vi "Draw_Grid_Over_Img.vi"(6 "[IN] Color":u32(colorbox)=16711680, 8 "error IN":errorcluster, 9 "[IN] Vertical step":i32=1 min=1 max=10000 step=1, 10 "[IN] Horiz step":i32=1 min=1 max=10000 step=1, 11 "[IN] Image":T1) -> (0 "error OUT":errorcluster, 3 "[OUT] Image":T1)   [LabVIEW 2020]
uses:
  <vilib>/vision/Image Controls.llb/IMAQ Image.ctl
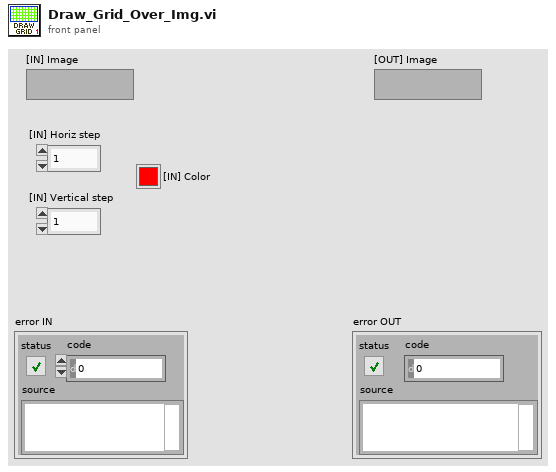
[diagram p1: front panel]
types:
  T1 = typedef "IMAQ Image.ctl" = refnum<image>
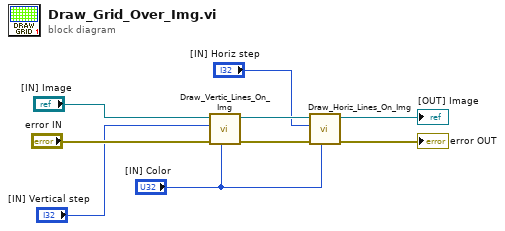
[diagram p0: block diagram]
diagram:
  n1 = call "Draw_Vertic_Lines_On_Img.vi"("[IN] Color"="[IN] Color", "error IN"="error IN", "[IN] Vertical step"="[IN] Vertical step", "[IN] Image"="[IN] Image") -> ("error OUT"=w6:errorcluster, "[OUT] Image"=w5:T1)  [unwired: 6 in]
  n2 = call "Draw_Horiz_Lines_On_Img.vi"("[IN] Color"="[IN] Color", "error IN"=w6, "[IN] Horizontal step"="[IN] Horiz step", "[IN] Image"=w5) -> ("error OUT"=→"error OUT":errorcluster, "[OUT] Image"=→"[OUT] Image":T1)  [unwired: 6 in]
